vi "WAM_UserBarCode_Popup.vi"(0 "Enable":bool=TRUE, 5 "error in (no error)":errorcluster) -> (10 "UserPromptInfo":string, 12 "operator infor header":string, 18 "OK":bool, 19 "error out":errorcluster)   [LabVIEW 2018]
doc: "Displays a standard dialog box that prompts users to enter information, such as a user name and password.\n--------------------\n\nThis Express VI is configured as follows:\n\nMessage to Display to the User:"
panel:
  in  "EmpLocation":string(combo) caption="LotID"
  in  "EmpName":string caption="Revision"
  in  "EmpID#":string caption="PN"
  out "String":string
  in  "Cancel":bool
  in  "OK2":bool
  in  "OK1":bool
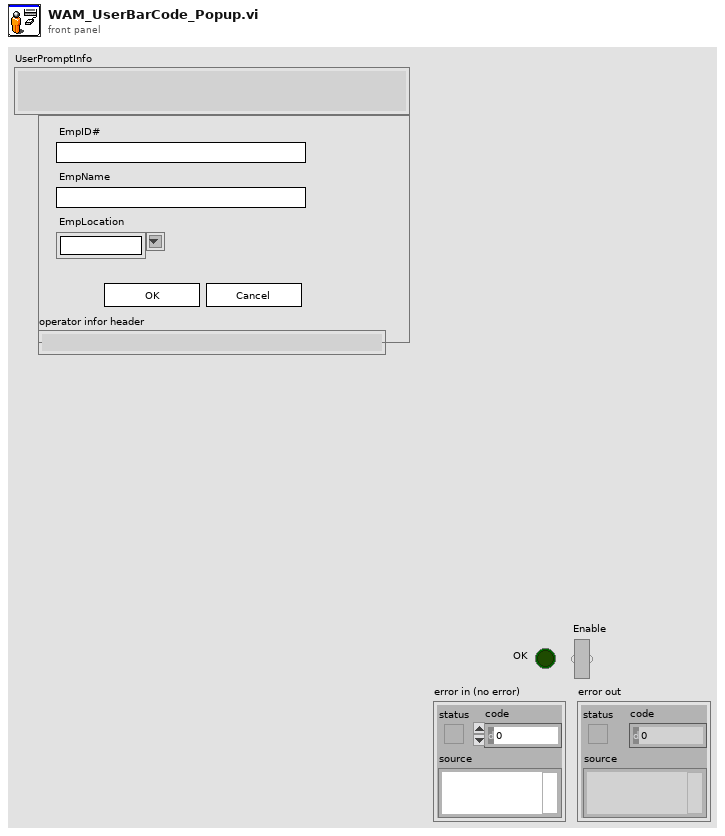
[diagram p1: front panel]
types:
  T1 = cluster{"Input Name":string, "Input Data Type":i32}[]
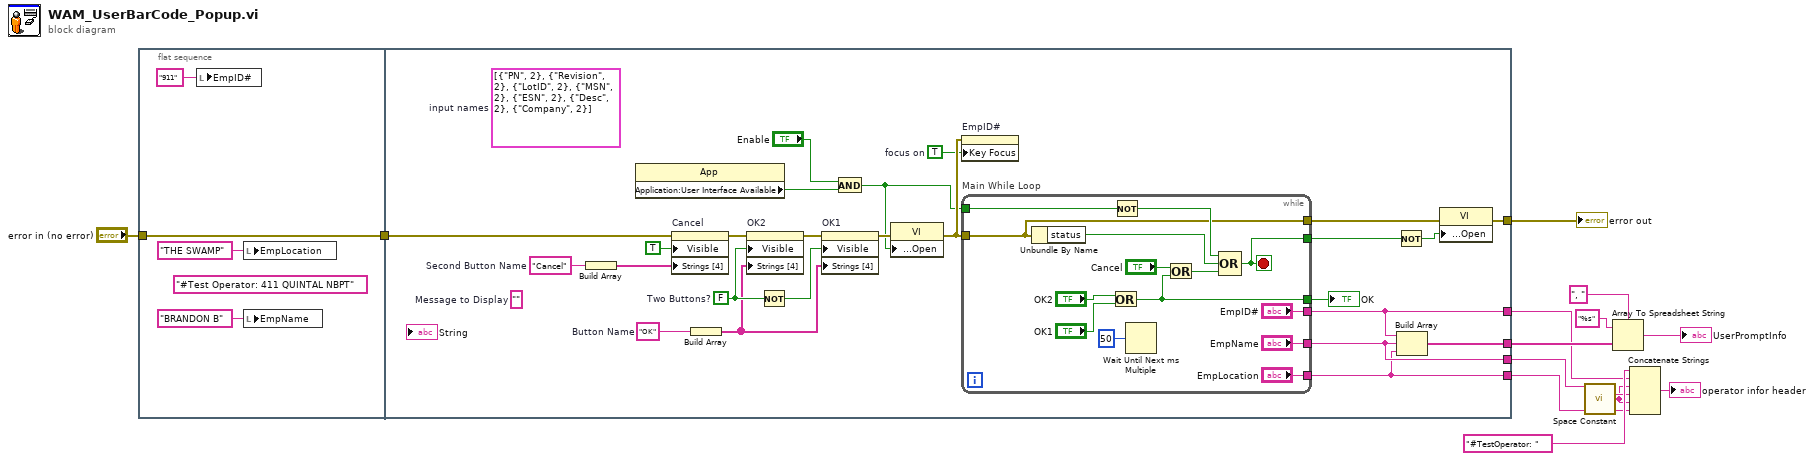
[diagram p0: block diagram]
diagram:
  n1 = flat-sequence {
    tunnel: "error in (no error)" -> [w17]
    tunnel: [w17] -> w7
    tunnel: [w27] -> w12
    tunnel: [w22] -> w11
    tunnel: w7 -> [w29]
    tunnel: [w20] -> w5
    tunnel: [w19] -> w4
    tunnel: [w18] -> w2
    frame #0 {
      (unwired) "#Test Operator: 411 QUINTAL NBPT" ("OperatorInfo")
      n2 = local write "EmpID#"("911" ("PN")) -> ()
      n3 = local write "EmpLocation"("THE SWAMP" ("LotID")) -> ()
      n4 = local write "EmpName"("BRANDON B" ("Revision")) -> ()
    }
    frame #1 {
      w23 = TRUE  # focus on
      (unwired) T1 [{"Input Name"="PN", "Input Data Type"=2}, {"Input Name"="Revision", "Input Data Type"=2}, {"Input Name"="LotID", "Input Data Type"=2}, {"Input Name"="MSN", "Input Data Type"=2}, {"Input Name"="ESN", "Input Data Type"=2}, {"Input Name"="Desc", "Input Data Type"=2}, {"Input Name"="Company", "Input Data Type"=2}]  # input names
      w34 = "Cancel"  # Second Button Name
      w32 = "OK"  # Button Name
      (unwired) ""  # Message to Display
      w42 = FALSE  # Two Buttons?
      n5 = Build Array(w34) -> (w35:string[])
      n6 = property class="App"() -> ("Application:User Interface Available"=w24:bool)  [unwired: 2 in, 2 out]
      n7 = property on="Cancel" class="Bool"(error in=w29, "Visible"=TRUE, "Strings [4]"=w35) -> (error out=w39:errorcluster)  [unwired: 1 in, 1 out]
      n8 = Build Array(w32) -> (w33:string[])
      n9 = property on="OK2" class="Bool"(error in=w39, "Visible"=w42, "Strings [4]"=w33) -> (error out=w38:errorcluster)  [unwired: 1 in, 1 out]
      n10 = Not(x=w42) -> (.not. x?=w40:bool)
      n11 = property on="OK1" class="Bool"(error in=w38, "Visible"=w40, "Strings [4]"=w33) -> (error out=w31:errorcluster)  [unwired: 1 in, 1 out]
      n12 = And(x="Enable", y=w24) -> (x .and. y?=w25:bool)
      n13 = property class="VI"(error in=w31, "Front Panel Window:Open"=w25) -> (error out=w30:errorcluster)  [unwired: 1 in, 1 out]
      n14 = property on="EmpID#" class="Str"(error in=w30, "Key Focus"=w23) -> ()  [unwired: 1 in, 2 out]
      n15 = while "Main While Loop" {
        tunnel: [w53] -> w41
        tunnel: w25 -> [w51]
        tunnel: [w49] -> w36
        tunnel: w30 -> [w48]
        tunnel: [w48] -> w28
        tunnel: ["EmpID#"] -> w20
        tunnel: ["EmpName"] -> w19
        tunnel: ["EmpLocation"] -> w18
        stop <- w49 stop-if-true
        n16 = Unbundle By Name(w48) -> ("status"=w46:bool)
        n17 = Or(x="OK2", y="OK1") -> (x .or. y?=w53:bool)
        n18 = Not(x=w51) -> (.not. x?=w50:bool)
        n19 = Wait Until Next ms Multiple(millisecond multiple=u32 50) -> ()  [unwired: 1 out]
        n20 = Or(x="Cancel", y=w53) -> (x .or. y?=w47:bool)
        n21 = Compound Arithmetic op=OR(w50, w46, w47) -> (w49:bool)
      }
      "OK" <- w41
      n22 = Not(x=w36) -> (.not. x?=w37:bool)
      n23 = Build Array(w20, w19, w18) -> (w22:string[])
      n24 = property class="VI"(error in=w28, "Front Panel Window:Open"=w37) -> (error out=w27:errorcluster)  [unwired: 1 in, 1 out]
    }
  }
  n25 = call <vilib>:"Space Constant.vi"() -> ("String"=w3:string)
  n26 = Array To Spreadsheet String(delimiter (Tab)=", ", array=w11, 3:"%s" ("format string")) -> (spreadsheet string=→"UserPromptInfo":string)
  n27 = Concatenate Strings("#TestOperator: " ("string"), w5, w3, w4, w3, w2) -> (→"operator infor header":string)
  "error out" <- w12
